vi "PicoScope6000ExampleRapidBlockBulk.vi"() -> ()   [LabVIEW 2009]
panel:
  in  "Trigger Settings":T1 {"Trigger Direction" items=["Rising", "Falling"]}
  in  "Channel A Settings":T2 {"Bandwidth" items=["Full", "20 MHz"]; "Range" items=["10 mV", "20 mV", "50 mV", "100 mV", "200 mV", "500 mV", "1 V", "2 V", "5 V", "10 V", "20 V", "50 V ", "100 V"]; "Coupling" items=["AC", "DC 1 MOhm", "DC 50 Ohm"]}
  in  "Rapid Block Acquisition Settings":T3
  out "Capture Complete":bool
  in  "Run":bool
  out "Channel A":i16[](graph)
  in  "Capture Index":i16 min=0
  in  "stop":bool
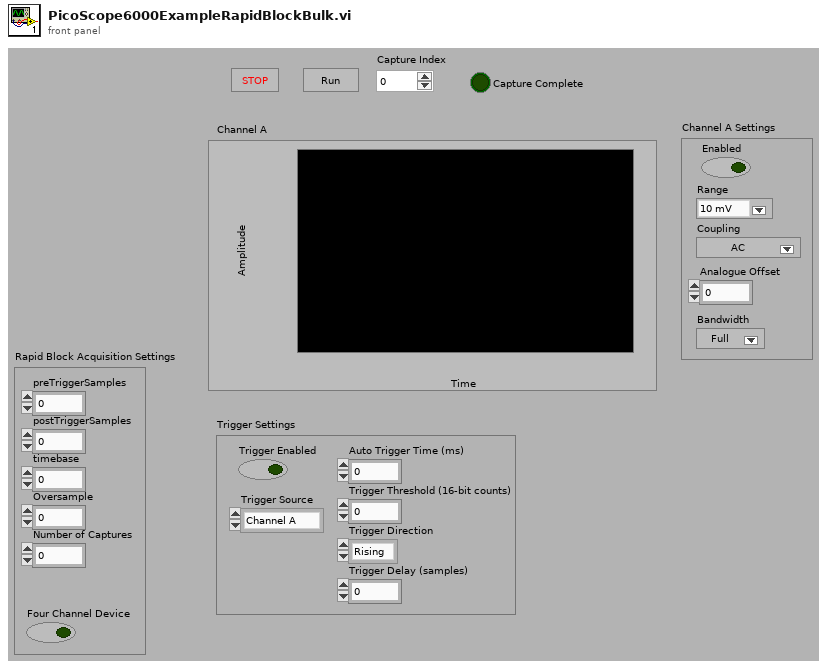
[diagram p1: front panel]
types:
  T1 = cluster{"Trigger Enabled":bool, "Trigger Source":enum32{"Channel A", "Channel B", "Channel C", "Channel D", "External", "Aux."}, "Trigger Threshold (16-bit counts)":i16, "Trigger Direction":u16, "Trigger Delay (samples)":u32, "Auto Trigger Time (ms)":i16}
  T2 = cluster{"Enabled":bool, "Coupling":u32, "Range":u32, "Analogue Offset":sgl, "Bandwidth":u32}
  T3 = cluster{"preTriggerSamples":u32, "postTriggerSamples":u32, "timebase":u32, "Four Channel Device":bool, "Oversample":i16, "Number of Captures":u32}
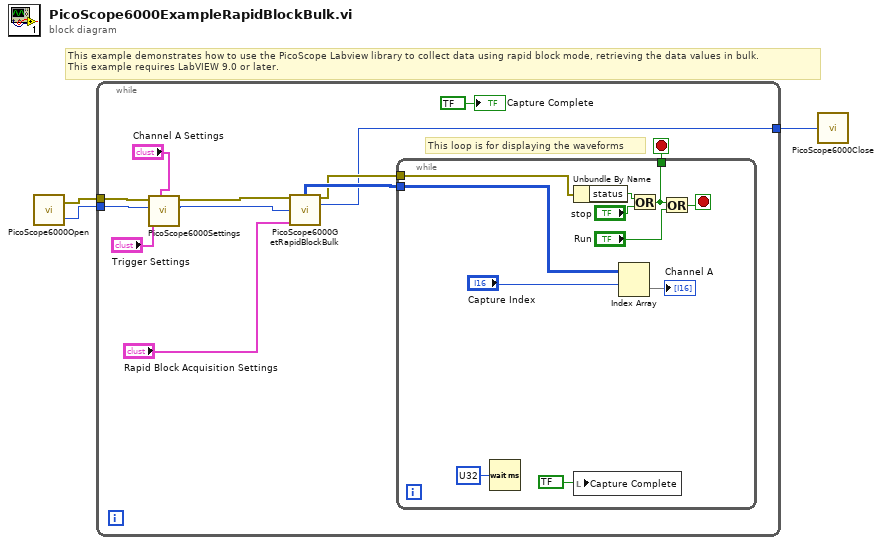
[diagram p0: block diagram]
diagram:
  # "This example demonstrates how to use the PicoScope Labview library to collect data using rapid block mode, retrieving the data values in bulk.\nThis example requires LabVIEW 9.0 or later."
  n1 = call "PicoScope6000Open.vi"() -> ("error out"=w2:errorcluster, "handle"=w1:i16)  [unwired: 1 in]
  n2 = while {
    tunnel: [w9] -> w3
    tunnel: w2 -> [w13]
    tunnel: w1 -> [w12]
    stop <- w15 stop-if-true
    # "This loop is for displaying the waveforms"
    n3 = call "PicoScope6000Settings.vi"("Channel A Settings"="Channel A Settings", "Trigger Settings"="Trigger Settings", "handle in"=w12, "error in"=w13) -> ("handle out"=w6:i16, "error out"=w7:errorcluster)  [unwired: 6 in]
    n4 = call "PicoScope6000GetRapidBlockBulk.vi"("error in"=w7, "handle in"=w6, "Rapid Block Acquisition Settings"="Rapid Block Acquisition Settings") -> ("Channel A Buffer"=w11:i16[][], "error out"=w10:errorcluster, "handle out"=w9:i16)  [unwired: 7 in, 3 out]
    n5 = while {
      tunnel: [w25] -> w15
      tunnel: w11 -> [w18]
      tunnel: w10 -> [w20]
      stop <- w24 stop-if-true
      n6 = Wait (ms)(milliseconds to wait=u32 ?) -> ()  [unwired: 1 out]
      n7 = Unbundle By Name(w20) -> ("status"=w19:bool)
      n8 = local write "Capture Complete"(bool ? ("Capture Complete")) -> ()
      n9 = Index Array(array=w18, index (row)="Capture Index") -> (element=→"Channel A":i16[])  [unwired: 1 in]
      n10 = Or(x=w19, y="stop") -> (x .or. y?=w25:bool)
      n11 = Or(x=w25, y="Run") -> (x .or. y?=w24:bool)
    }
    "Capture Complete" <- bool ? ("Capture Complete")
  }
  n12 = call "PicoScope6000Close.vi"("handle"=w3) -> ()
